vi "Enable Measurements.vi"(0 "Register Buses":refnum<class "ni579x Register Bus v1 Host.lvclass">[](array[class]), 9 "timeout (s) (10)":dbl=10.0, 11 "error in":errorcluster) -> (4 "Register Buses (out)":refnum<class "ni579x Register Bus v1 Host.lvclass">[](array[class]), 15 "error out":errorcluster)   [LabVIEW 2012, in "ni579x Synchronization v1 Host.lvlib"]
doc: "Turn on the measurement circuits on the FPGA. This also involves setting the master, which will be the first FPGA in the array of FPGA VI References."
uses:
  <instrlib>/ni579x/Synchronization/v1/Host/ni579x Synchronization v1 Host.lvlib
  <instrlib>/ni579x/Register Bus/v1/Host/ni579x Register Bus v1 Host.lvclass
  <instrlib>/ni579x/Synchronization/v1/Shared/ni579x Synchronization Register Addresses.ctl
  <instrlib>/ni579x/Register Bus/v1/Host/Public/Register Write.ctl
  <instrlib>/ni579x/Config/v1/Shared/Types/ni579x Register Bus Subsystem ID.ctl
  <instrlib>/ni579x/Register Bus/v1/Host/Public/Register Read Request.ctl
  <vilib>/Utility/error.llb/Error Cluster From Error Code.vi
  <vilib>/ErrorRing/Error Ring.xnode
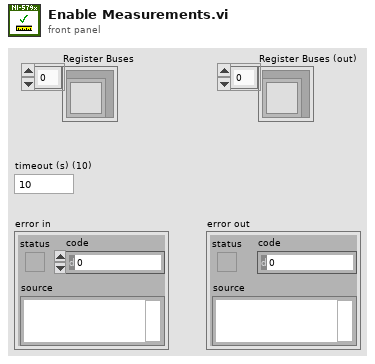
[diagram p1: front panel]
types:
  T1 = typedef "ni579x Register Bus v1 Host.lvclass/Register Read Request.ctl" = cluster{"subsystem":u8, "address":u16}
  T2 = typedef "ni579x Register Bus Subsystem ID.ctl" = u8
  T3 = typedef "ni579x Synchronization Register Addresses.ctl" = enum16{"Signature", "Current Version", "Oldest Compatible Version", "Scratch Register", "sync.master", "sync.meas.enable", "sync.meas.ready", "sync.meas.arm", "sync.meas.valid", "sync.meas.value", "sync.cptr.adjust", "sync.cptr.period", "sync.meas.oversample factor"}
  T4 = typedef "ni579x Register Bus v1 Host.lvclass/Register Write.ctl" = cluster{"subsystem":u8, "address":u16, "data":u32}
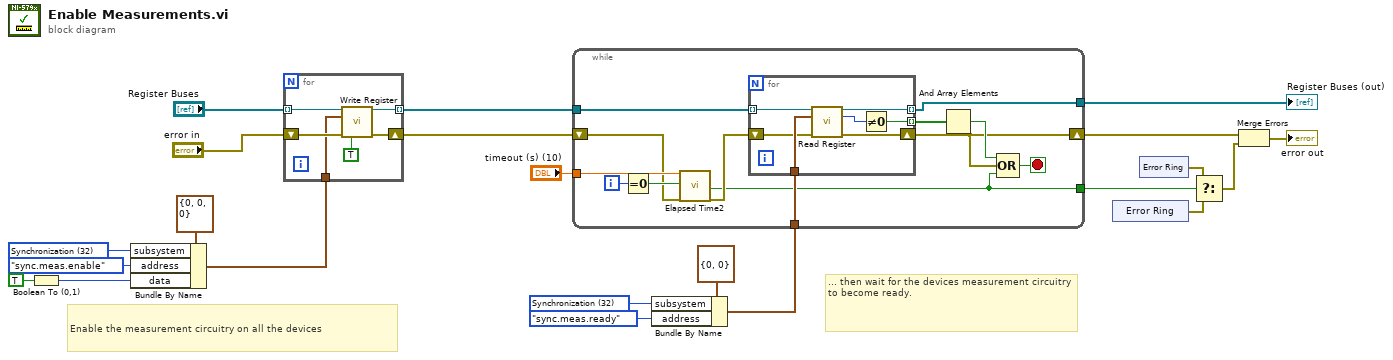
[diagram p0: block diagram]
diagram:
  w10 = T2 32 items=["FAM Register Operation"=0, "User Command"=16, "Synchronization"=32] ("Subsystem ID")
  w16 = T2 32 items=["FAM Register Operation"=0, "User Command"=16, "Synchronization"=32] ("Subsystem ID")
  # "... then wait for the devices measurement circuitry to become ready."
  # "Enable the measurement circuitry on all the devices"
  n1 = Boolean To (0,1)(Boolean=TRUE ("sync.Master")) -> (0, 1=w18:i16)
  n2 = Bundle By Name(cluster=T4 {"subsystem"=0, "address"=0, "data"=0} ("register write"), "subsystem"=w16, "address"=ni579x_Synchronization_Register_Addresses."sync.meas.enable" ("Synchronization Registers"), "data"=w18) -> (w13:T4)
  n3 = for {
    tunnel: "Register Buses" -> [w28] mode=indexing
    tunnel: w13 -> [w26]
    tunnel: [w24] -> w5 mode=indexing
    shift-right: [w23] -> w4
    shift-left: "error in" -> [w27]
    n4 = call <instrlib>:"Write Register.vi"("session in"=w28, "register write"=w26, "error in"=w27, "wait until committed"=TRUE) -> ("session out"=w24:refnum<class "ni579x Register Bus v1 Host.lvclass">, "error out"=w23:errorcluster)  [unwired: 10 in]
  }
  n5 = Bundle By Name(cluster=T1 {"subsystem"=0, "address"=0} ("register read request"), "subsystem"=w10, "address"=ni579x_Synchronization_Register_Addresses."sync.meas.ready" ("Synchronization Registers")) -> (w8:T1)
  n6 = while {
    tunnel: w8 -> [w41]
    tunnel: "timeout (s) (10)" -> [w38]
    tunnel: w5 -> [w36]
    shift-right: [w32] -> w3
    shift-left: w4 -> [w35]
    tunnel: [w30] -> w2
    tunnel: [w29] -> w1
    i -> [w39]
    stop <- w31 stop-if-true
    n7 = Equal To 0?(x=w39) -> (x = 0?=w40:bool)
    n8 = call "Elapsed Time2"("Time Target (s)"=w38, "Reset"=w40, "error in (no error)"=w35) -> ("Time has Elapsed"=w30:bool, "error out"=w37:errorcluster)  [unwired: 9 in, 6 out]
    n9 = for {
      tunnel: w41 -> [w48]
      shift-right: [w45] -> w32
      shift-left: w37 -> [w46]
      tunnel: w36 -> [w44] mode=indexing
      tunnel: [w43] -> w34 mode=indexing
      tunnel: [w42] -> w29 mode=indexing
      n10 = call <instrlib>:"Read Register.vi"("session in"=w44, "register read request"=w48, "error in"=w46) -> ("session out"=w42:refnum<class "ni579x Register Bus v1 Host.lvclass">, "data"=w47:u32, "error out"=w45:errorcluster)  [unwired: 10 in]
      n11 = Not Equal To 0?(x=w47) -> (x != 0?=w43:bool)
    }
    n12 = And Array Elements(Boolean array=w34) -> (logical AND=w33:bool)
    n13 = Compound Arithmetic op=OR(w33, w32, w30) -> (w31:bool)
  }
  "Register Buses (out)" <- w1
  n14 = xnode "Error Ring"() -> ("error out"=w20:errorcluster)
  n15 = xnode "Error Ring"() -> ("error out"=w19:errorcluster)
  n16 = Select(t=w19, s=w2, f=w20) -> (s? t:f=w22:errorcluster)
  n17 = Merge Errors(w3, w22) -> (→"error out":errorcluster)
